vi "Configure Edge Trigger Source.vi"(0 "VISA resource name":refnum<visa-resource-name>, 5 "Trigger Source (0: Channel 1)":u16(ring) items=["Channel 1", "Channel 2", "Channel 3", "Channel 4", "DIG 0", "DIG 1", "DIG 2", "DIG 3", "DIG 4", "DIG 5", "DIG 6", "DIG 7", "DIG 8", "DIG 9", "DIG 10", "DIG 11", "DIG 12", "DIG 13", "DIG 14", "DIG 15", "Line", "External"], 7 "Trigger Slope (0: Positive)":u16(ring) items=["Positive", "Negative", "Either", "Alternate"], 9 "Trigger Level (0.0 V)":dbl, 11 "error in (no error)":errorcluster) -> (4 "VISA resource name out":refnum<visa-resource-name>, 15 "error out":errorcluster)   [LabVIEW 2017, in "Agilent 6000 Series.lvlib"]
doc: "Configures edge trigger settings. An edge trigger occurs when the trigger signal passes through the voltage threshold that you specify with the Level control and has the slope that you specify with the Slope control."
uses:
  <instrlib>/Agilent 6000 Series/Agilent 6000 Series.lvlib
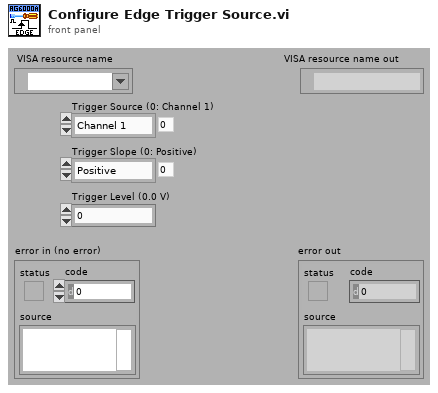
[diagram p1: front panel]
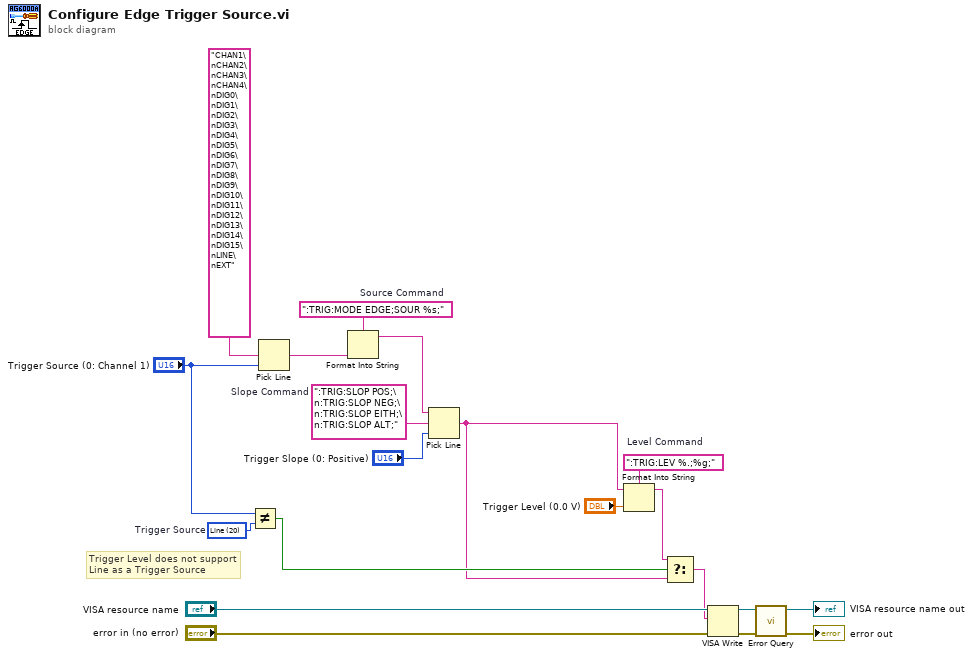
[diagram p0: block diagram]
diagram:
  w7 = u16 20 items=["Channel 1", "Channel 2", "Channel 3", "Channel 4", "DIG 0", "DIG 1", "DIG 2", "DIG 3", "DIG 4", "DIG 5", "DIG 6", "DIG 7", "DIG 8", "DIG 9", "DIG 10", "DIG 11", "DIG 12", "DIG 13", "DIG 14", "DIG 15", "Line", "External"]  # Trigger Source
  w10 = ":TRIG:SLOP POS;\n:TRIG:SLOP NEG;\n:TRIG:SLOP EITH;\n:TRIG:SLOP ALT;"  # Slope Command
  w13 = ":TRIG:LEV %.;%g;"  # Level Command
  w14 = ":TRIG:MODE EDGE;SOUR %s;"  # Source Command
  # "Trigger Level does not support \nLine as a Trigger Source"
  n1 = Not Equal?(x="Trigger Source (0: Channel 1)", y=w7) -> (x != y?=w4:bool)
  n2 = Pick Line(multi-line string="CHAN1\nCHAN2\nCHAN3\nCHAN4\nDIG0\nDIG1\nDIG2\nDIG3\nDIG4\nDIG5\nDIG6\nDIG7\nDIG8\nDIG9\nDIG10\nDIG11\nDIG12\nDIG13\nDIG14\nDIG15\nLINE\nEXT", line index="Trigger Source (0: Channel 1)") -> (output string=w6:string)  [unwired: 1 in]
  n3 = Format Into String(format string=w14, w6) -> (resulting string=w8:string)  [unwired: 2 in, 1 out]
  n4 = Pick Line(string ("")=w8, multi-line string=w10, line index="Trigger Slope (0: Positive)") -> (output string=w2:string)
  n5 = Format Into String(format string=w13, initial string=w2, "Trigger Level (0.0 V)") -> (resulting string=w3:string)  [unwired: 1 in, 1 out]
  n6 = Select(t=w3, s=w4, f=w2) -> (s? t:f=w1:string)
  n7 = VISA Write(VISA resource name="VISA resource name", write buffer=w1, error in (no error)="error in (no error)") -> (VISA resource name out=w16:refnum<visa-resource-name>, error out=w15:errorcluster)  [unwired: 1 out]
  n8 = call <instrlib>:"Error Query.vi"("error in (no error)"=w15, "VISA resource name"=w16) -> ("error out"=→"error out":errorcluster, "VISA resource name out"=→"VISA resource name out":refnum<visa-resource-name>)  [unwired: 6 in, 2 out]
